vi "Utility - ICPCON.vi"(8 "error in":errorcluster caption="错误输入（无错误）", 11 "VISA resource name":refnum<visa-resource-name>="COM1") -> (0 "error out":errorcluster caption="错误输出", 3 "Measurement Data":sgl[](array[numeric]) caption="测量数据" format="%.2g")   [LabVIEW 2015]
uses:
  <vilib>/Instr/_visa.llb/VISA Configure Serial Port (Instr).vi
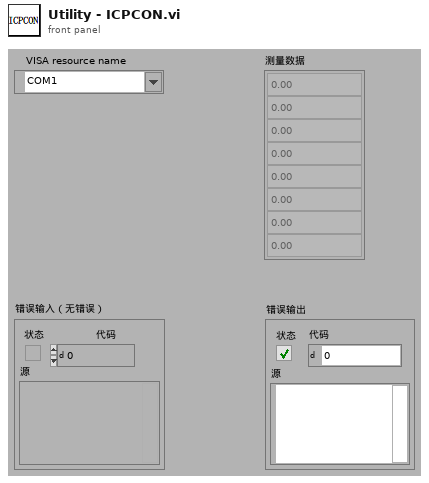
[diagram p1: front panel]
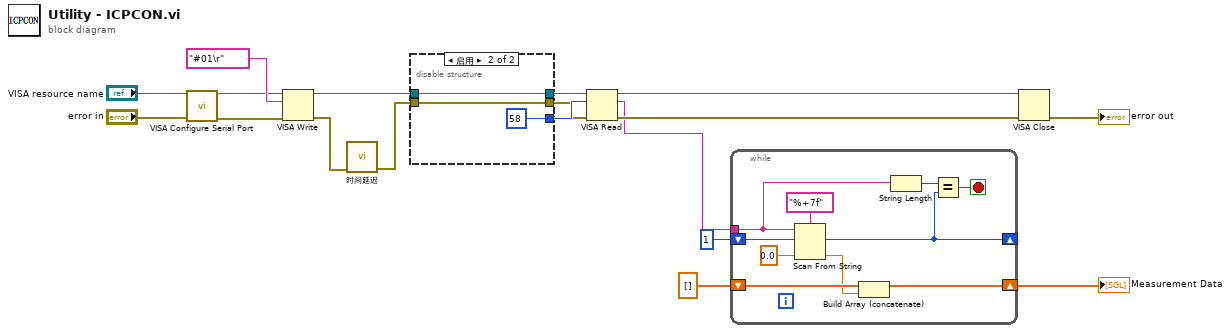
[diagram p0: block diagram]
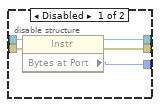
[diagram p2: hidden frame]
diagram:
  n1 = call-poly "VISA Configure Serial Port"("VISA resource name"="VISA resource name", "error in (no error)"="error in") -> ("VISA resource name out"=w8:refnum<visa-resource-name>, "error out"=w5:errorcluster)  [unwired: 12 in]
  n2 = VISA Write(VISA resource name=w8, write buffer="#01\r" ("写入缓冲区"), error in (no error)=w5) -> (VISA resource name out=w15:refnum<visa-resource-name>, error out=w12:errorcluster)  [unwired: 1 out]
  n3 = call "时间延迟"("error in (no error)"=w12) -> ("error out"=w10:errorcluster)  [unwired: 10 in]
  n4 = disable-structure shown="启用" {
    disable-tunnel: w15 -> [w23 w26]
    disable-tunnel: [w22 w26] -> w14
    disable-tunnel: [w21 u32 58 ("Bytes at Port")] -> w13
    disable-tunnel: [w20 w25] -> w11
    disable-tunnel: w10 -> [w19 w25]
    frame Disabled {
      n5 = property class="Instr"(reference=w23, error in=w19) -> (reference out=w22:refnum<visa-resource-name>, error out=w20:errorcluster, "Bytes at Port"=w21:u32)
    }
    frame Enabled {
    }
  }
  n6 = VISA Read(VISA resource name=w14, byte count=w13, error in (no error)=w11) -> (VISA resource name out=w17:refnum<visa-resource-name>, read buffer=w2:string, error out=w16:errorcluster)  [unwired: 1 out]
  n7 = while {
    shift-right: [w35] -> w3
    shift-left: sgl[] [] -> [w34]
    shift-right: [w28] -> _
    shift-left: u32 1 -> [w29]
    tunnel: w2 -> [w27]
    stop <- w31 stop-if-true
    n8 = Scan From String(format string="%+7f", input string=w27, initial scan location=w29, default 1=sgl 0.0 ("default value 1")) -> (offset past scan=w28:u32, output 1=w33:sgl)  [unwired: 1 in, 2 out]
    n9 = Build Array (concatenate)(w34, w33) -> (w35:sgl[])
    n10 = String Length(string=w27) -> (length=w32:i32)
    n11 = Equal?(x=w32, y=w28) -> (x = y?=w31:bool)
  }
  "Measurement Data" <- w3
  n12 = VISA Close(VISA resource name=w17, error in (no error)=w16) -> (error out=→"error out":errorcluster)
